vi "AI增加一条自动检测记录.vi"(8 "测试结果":string, 10 "最大误差":dbl, 11 "测试内容":string) -> ()   [LabVIEW 2010]
uses:
  全局量/自动测试结果.vi
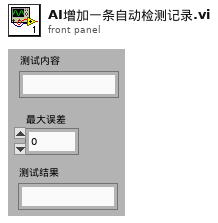
[diagram p1: front panel]
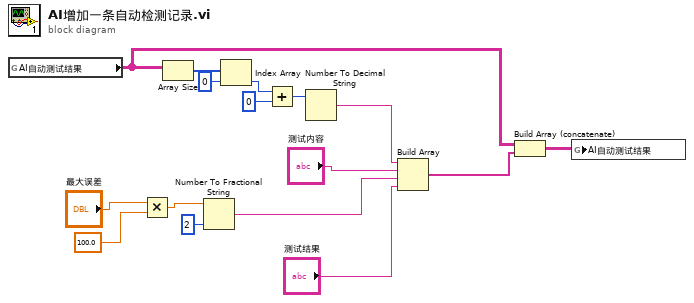
[diagram p0: block diagram]
diagram:
  n1 = global read "自动测试结果.vi" "AI自动测试结果"() -> (w9:string[][])
  n2 = Multiply(x="最大误差", y=100.0) -> (x*y=w2:dbl)
  n3 = Array Size(array=w9) -> (size(s)=w16:i32[])
  n4 = Number To Fractional String(number=w2, precision (6)=i16 2 ("精度(6)")) -> (F-format string=w5:string)  [unwired: 2 in]
  n5 = Index Array(array=w16, index=0 ("索引")) -> (element=w14:i32)
  n6 = Add(x=w14, y=0) -> (x+y=w12:i32)
  n7 = Number To Decimal String(number=w12) -> (decimal integer string=w11:string)  [unwired: 1 in]
  n8 = Build Array(w11, "测试内容", w5, "测试结果") -> (w8:string[])
  n9 = Build Array (concatenate)(w9, w8) -> (w7:string[][])
  n10 = global write "自动测试结果.vi" "AI自动测试结果"(w7) -> ()
